vi "Save OPC Configuration.vi"(8 "Error In":errorcluster, 10 "OPC Settings":T1={"OPC Server Endpoint URL"="opc.tcp://XPS15HPH:49580", "OPC Node Id"="ns=2;s=ProcessData.Temperature"}) -> (0 "Error Out":errorcluster)   [LabVIEW 2018]
uses:
  <vilib>/Utility/config.llb/Write Key (String).vi
  <vilib>/Utility/config.llb/NI_LVConfig.lvlib
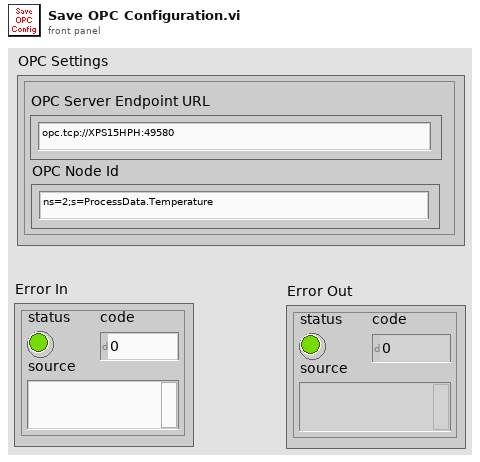
[diagram p1: front panel]
types:
  T1 = cluster{"OPC Server Endpoint URL":string, "OPC Node Id":string}
  T2 = typedef "NI_LVConfig.lvlib/Config Data RefNum.ctl" = refnum<k1>
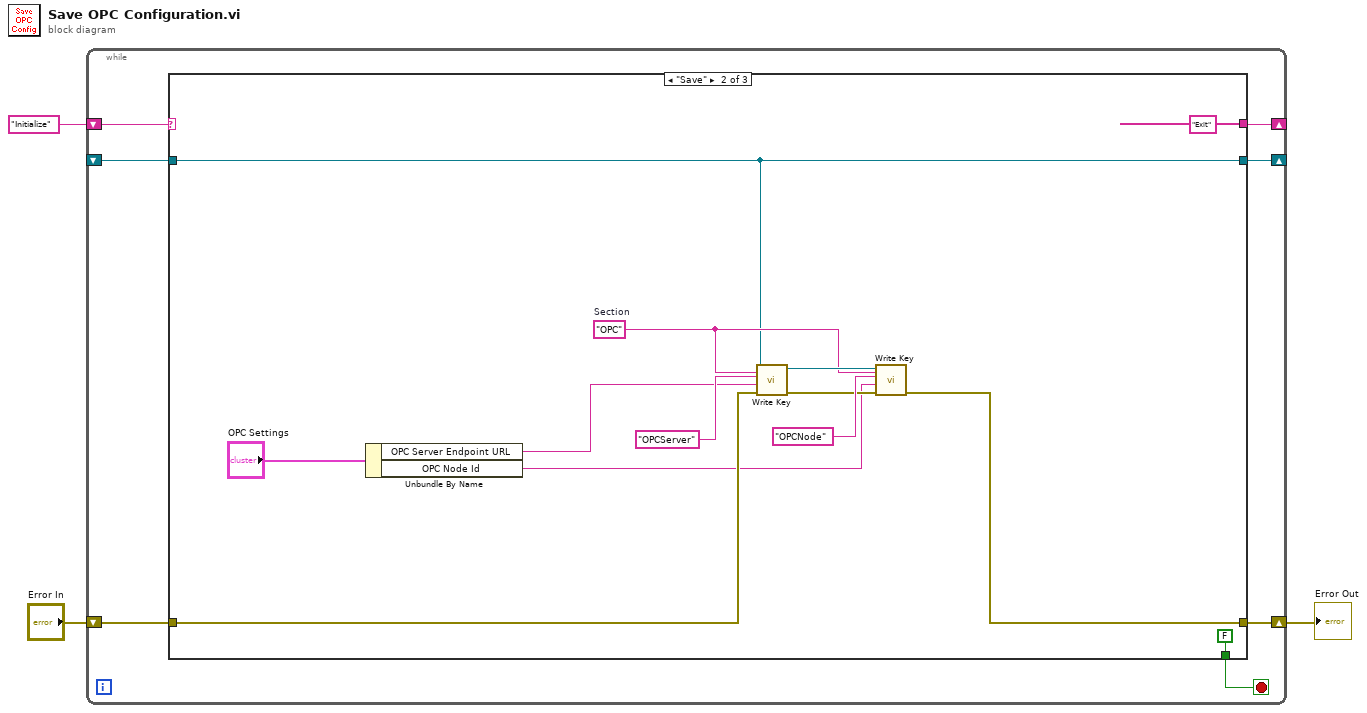
[diagram p0: block diagram]
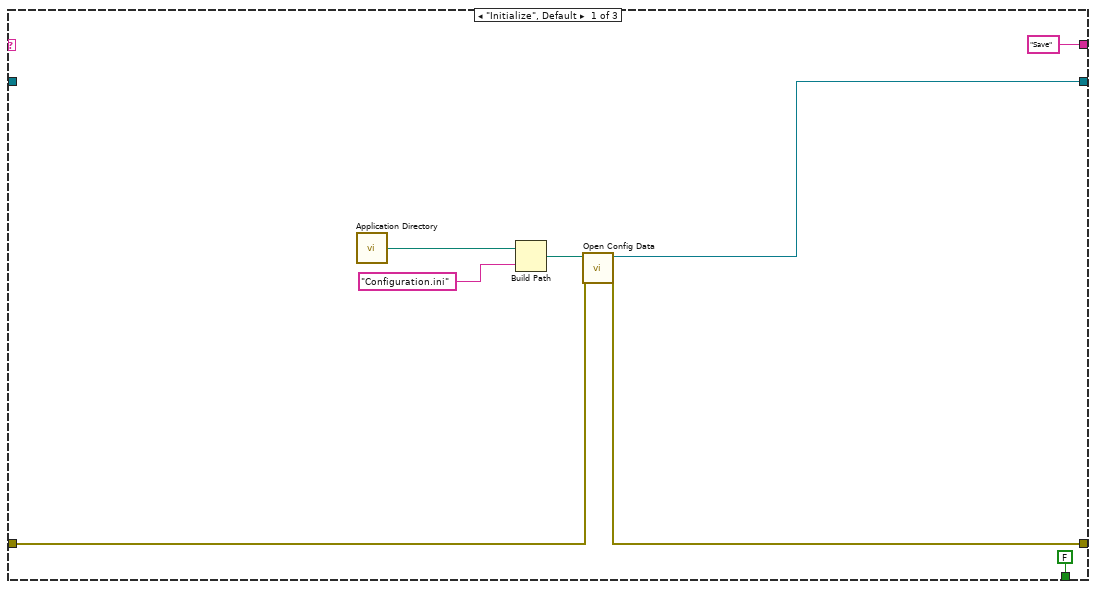
[diagram p2: hidden frame]
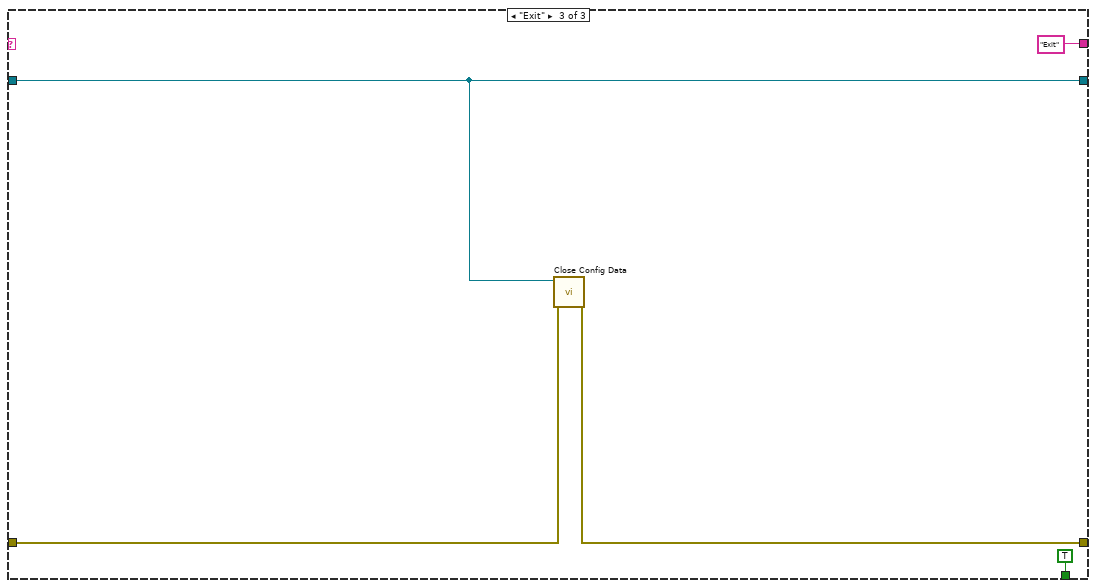
[diagram p3: hidden frame]
diagram:
  n1 = while {
    shift-right: [w6] -> _
    shift-left: "Initialize" ("key") -> [w10]
    shift-right: [w7] -> _
    shift-left: _ -> [w9]
    shift-right: [w4] -> w1
    shift-left: "Error In" -> [w8]
    stop <- w5 stop-if-true
    n2 = case shown="\"Save\"" w10 {
      tunnel: w9 -> [_ w19 w34]
      tunnel: w8 -> [w12 w24 w33]
      tunnel: [w13 w19 w34] -> w7
      tunnel: ["Save" ("key") "Exit" ("key") "Exit" ("key")] -> w6
      tunnel: [FALSE FALSE TRUE] -> w5
      tunnel: [w11 w20 w32] -> w4
      frame "Initialize", Default {
        n3 = call <vilib>:"Application Directory.vi"() -> ("Application Directory"=w16:path)
        n4 = Build Path(base path=w16, name or relative path="Configuration.ini") -> (appended path=w14:path)
        n5 = call <vilib>:"Open Config Data.vi"("error in (no error)"=w12, "configuration file path"=w14) -> ("error out"=w11:errorcluster, "refnum"=w13:T2)  [unwired: 7 in, 1 out]
      }
      frame "Save" {
        w25 = "OPC"  # Section
        n6 = Unbundle By Name("OPC Settings") -> ("OPC Server Endpoint URL"=w22:string, "OPC Node Id"=w21:string)
        n7 = call-poly <vilib>:"Write Key.vi"("section"=w25, "error in (no error)"=w24, "value"=w22, "key"="OPCServer", "refnum"=w19) -> ("error out"=w28:errorcluster, "refnum out"=w27:T2)  [unwired: 4 in, 1 out]
        n8 = call-poly <vilib>:"Write Key.vi"("section"=w25, "error in (no error)"=w28, "value"=w21, "key"="OPCNode", "refnum"=w27) -> ("error out"=w20:errorcluster)  [unwired: 4 in, 2 out]
      }
      frame "Exit" {
        n9 = call <vilib>:"Close Config Data.vi"("error in (no error)"=w33, "refnum"=w34) -> ("error out"=w32:errorcluster)  [unwired: 8 in, 1 out]
      }
    }
  }
  "Error Out" <- w1
